vi "test Scheduled Loopback on Same Core.vi"(8 "error in":errorcluster, 11 "TestCase in":refnum<class "Multiple Instances.lvclass">) -> (0 "error out":errorcluster, 3 "TestCase out":refnum<class "Multiple Instances.lvclass">)   [LabVIEW 2020, in "Multiple Instances.lvclass"]
uses:
  Multiple Instances.lvclass
  C:/Program Files (x86)/National Instruments/LabVIEW 2020/vi.lib/NI/VeriStand Custom Device Testing Tools/VeriStandTestCase/VeriStandTestCase.lvclass
  <vilib>/NI VeriStand/Execution/Workspace/NI VeriStand - Get Single Channel Value.vi
  <vilib>/addons/_JKI Toolkits/VI Tester/TestCase.llb/TestCase.lvclass
  <vilib>/NI/VeriStand Custom Device Testing Tools/VeriStandTestUtilities/VeriStandTestUtilities.lvlib
  <vilib>/NI VeriStand/Execution/Workspace/NI_VS Workspace ExecutionAPI.lvlib
  C:/Program Files (x86)/National Instruments/LabVIEW 2020/vi.lib/addons/_JKI Toolkits/VI Tester/TestCase.llb/TestCase.lvclass
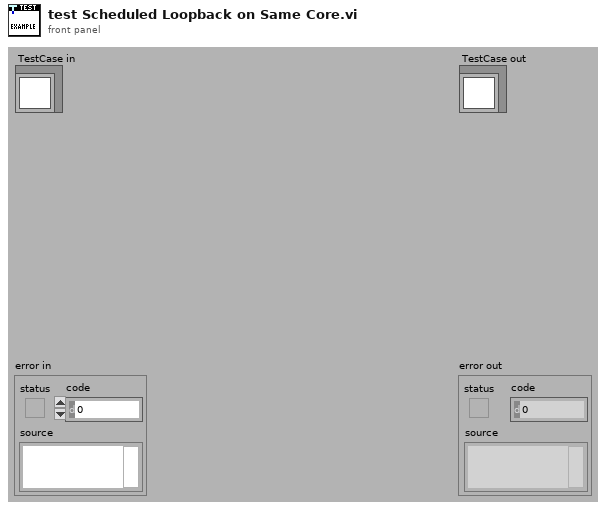
[diagram p1: front panel]
types:
  T1 = typedef "NI_VS Workspace ExecutionAPI.lvlib/WorkspaceAPI.ctl" = refnum<k24>
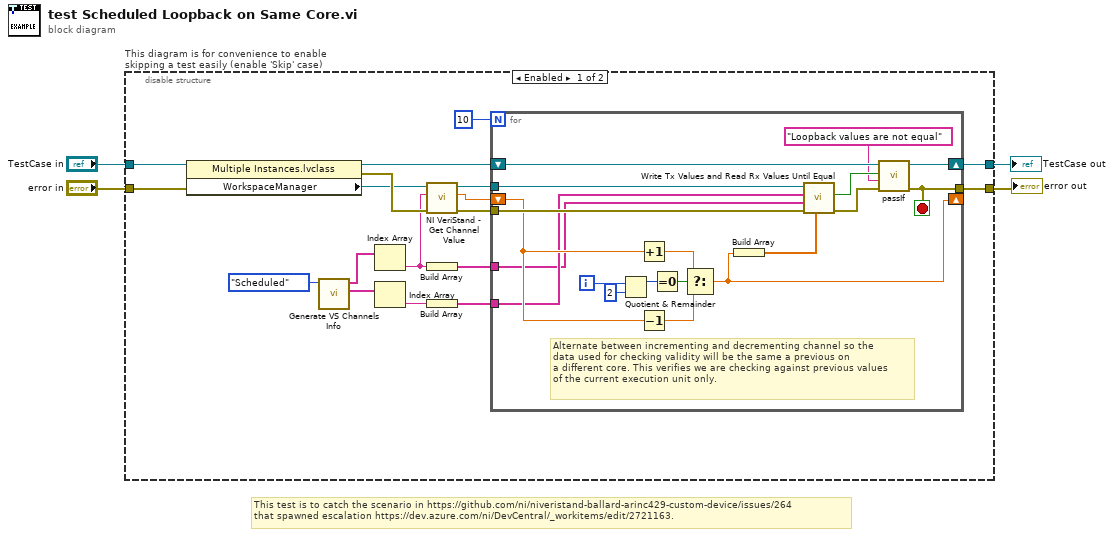
[diagram p0: block diagram]
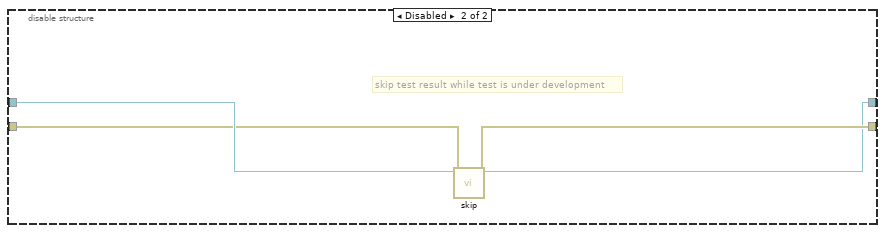
[diagram p2: hidden frame]
diagram:
  # "This test is to catch the scenario in https://github.com/ni/niveristand-ballard-arinc429-custom-device/issues/264\nthat spawned escalation https://dev.azure.com/ni/DevCentral/_workitems/edit/2721163."
  n1 = disable-structure "This diagram is for convenience to enable skipping a test easily (enable 'Skip' case)" shown="Enabled" {
    disable-tunnel: "TestCase in" -> [w19 w45]
    disable-tunnel: [w16 w43] -> w1
    disable-tunnel: [w17 w44] -> w3
    disable-tunnel: "error in" -> [w18 w42]
    frame Enabled {
      n2 = property class="Multiple Instances.lvclass"(reference=w19, error in=w18) -> (reference out=w22:refnum<class "Multiple Instances.lvclass">, error out=w15:errorcluster, "WorkspaceManager"=w14:T1)
      n3 = call "Generate VS Channels Info.vi"("Transfer Type"=enum16{"Acyclic", "Scheduled"}."Scheduled") -> ("Tx Channels Array"=w9:string[], "Rx Channels Array"=w11:string[])  [unwired: 6 in, 3 out]
      n4 = Index Array(array=w11) -> (element=w8:string)  [unwired: 1 in]
      n5 = Index Array(array=w9) -> (element=w7:string)  [unwired: 1 in]
      n6 = call-poly <vilib>:"NI VeriStand - Get Channel Value.vi"("error in (no error)"=w15, "Channel"=w8, "WorkspaceManager in"=w14) -> ("error out"=w12:errorcluster, "Value"=w10:dbl, "WorkspaceManager out"=w13:T1)  [unwired: 6 in]
      n7 = Build Array(w8) -> (w6:string[])
      n8 = Build Array(w7) -> (w5:string[])
      n9 = for {
        N: 10 -> [_]
        tunnel: w13 -> [w41]
        tunnel: w12 -> [w40]
        shift-right: [w37] -> w16
        shift-left: w22 -> [w38]
        tunnel: [w36] -> w17
        shift-right: [w25] -> _
        shift-left: w10 -> [w29]
        tunnel: w6 -> [w23]
        tunnel: w5 -> [w24]
        i -> [w33]
        stop <- w36 stop-if-true
        # "Alternate between incrementing and decrementing channel so the\ndata used for checking validity will be the same a previous on\na different core. This verifies we are checking against previous values\nof the current execution unit only."
        n10 = Quotient & Remainder(x=w33, y=2) -> (x-y*floor(x/y)=w31:i32)  [unwired: 1 out]
        n11 = Increment(x=w29) -> (x+1=w28:dbl)
        n12 = Decrement(x=w29) -> (x-1=w27:dbl)
        n13 = Equal To 0?(x=w31) -> (x = 0?=w30:bool)
        n14 = Select(t=w28, s=w30, f=w27) -> (s? t:f=w25:dbl)
        n15 = Build Array(w25) -> (w26:dbl[])
        n16 = call <vilib>:"Write Tx Values and Read Rx Values Until Equal.vi"("Tx values"=w26, "error in"=w40, "Rx aliases"=w23, "Tx aliases"=w24, "workspace manager in"=w41) -> ("error out"=w39:errorcluster, "values equal"=w35:bool)  [unwired: 4 in, 1 out]
        n17 = call-dynamic "passIf.vi"("error in (no error)"=w39, "message (\"\")"="Loopback values are not equal" ("message (\"\")"), "pass"=w35, "TestCase in"=w38) -> ("error out"=w36:errorcluster, "TestCase out"=w37:refnum<class "Multiple Instances.lvclass">)  [unwired: 6 in]
      }
    }
    frame Disabled {
      # "skip test result while test is under development"
      n18 = call <vilib>:"skip.vi"("error in (no error)"=w42, "TestCase in"=w45) -> ("error out"=w44:errorcluster, "TestCase out"=w43:refnum<class "Multiple Instances.lvclass">)  [unwired: 8 in]
    }
  }
  "error out" <- w3
  "TestCase out" <- w1
